vi "channel.description.vi"(8 "error in":errorcluster, 11 "Channel in":refnum<class "Channel.lvclass">) -> (0 "error out":errorcluster, 2 "description":string, 3 "Channel out":refnum<class "Channel.lvclass">)   [LabVIEW 2020, in "Channel.lvclass"]
doc: "Returns the channel's description, if one is set."
uses:
  Channel.lvclass
  Channel.lvclass/Channel.ctl
  client.lvlib
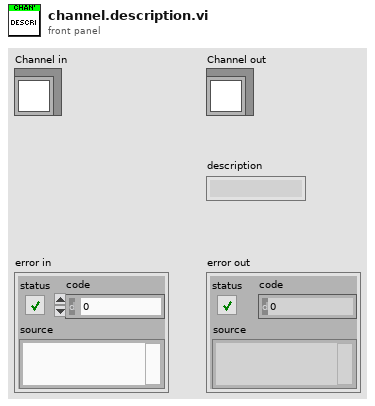
[diagram p1: front panel]
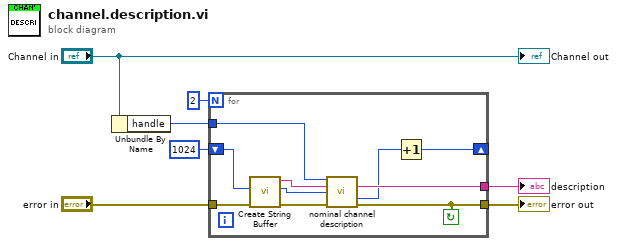
[diagram p0: block diagram]
diagram:
  n1 = Unbundle By Name("Channel in") -> ("handle"=w4:i32)
  n2 = for {
    N: 2 -> [_]
    tunnel: w4 -> [w17]
    tunnel: [w16] -> w1
    shift-right: [w8] -> _
    shift-left: 1024 ("Buffer Size (1024)") -> [w13]
    tunnel: "error in" -> [w11]
    tunnel: [w9] -> w2
    stop <- w9 continue-if-true
    n3 = call "Create String Buffer.vi"("error in"=w11, "Buffer Size (1024)"=w13) -> ("error out"=w12:errorcluster, "dub Buffer Size"=w14:i32, "String Buffer"=w15:string)  [unwired: 7 in]
    n4 = call "nominal channel description.vi"("channel"=w17, "buf"=w15, "cap"=w14, "error in (no error)"=w12) -> ("buf out"=w16:string, "out_needed out"=w10:u32, "error out"=w9:errorcluster)  [unwired: 7 in, 2 out]
    n5 = Increment(x=w10) -> (x+1=w8:u32)
  }
  "error out" <- w2
  "description" <- w1
  "Channel out" <- "Channel in"
